vi "Pre Launch Init.vi"(11 "UserInterface in":refnum<class "UserInterface.lvclass">) -> (0 "error out":errorcluster, 3 "UserInterface out":refnum<class "UserInterface.lvclass">)   [LabVIEW 2022 SP3, in "UserInterface.lvlib" / "UserInterface.lvclass"]
doc: "(<B>Filename</B>: Actor Framework.lvlib:Actor.lvclass:Pre Launch Init.vi)\n\nDefines behavior that occurs after the Launch Nested Actor method is invoked but before the actor's Actor Core method begins running.\n\nBy default, this method does nothing. A descendant class may override it to define behavior."
uses:
  UserInterface.lvclass
  <vilib>/ActorFramework/Actor/Actor.lvclass
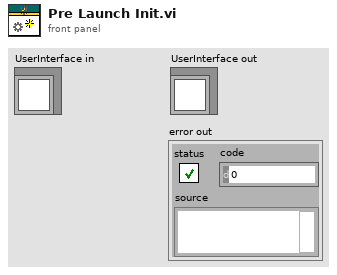
[diagram p1: front panel]
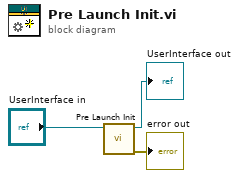
[diagram p0: block diagram]
diagram:
  n1 = call-parent "Pre Launch Init.vi"("Actor in"="UserInterface in") -> ("error out"=→"error out":errorcluster, "Actor out"=→"UserInterface out":refnum<class "UserInterface.lvclass">)  [unwired: 9 in]
